vi "LocalHostServer.vi"() -> ()   [LabVIEW 2016]
uses:
  FTT/controls/SocketServerStates.ctl
panel:
  out "LocalHostCommState":bool
  out "Ch2":fxp<+/-,20,5>
  out "Ch1":fxp<+/-,20,5>
  out "error out":errorcluster
  in  "error in (no error)":errorcluster
  in  "stop":bool
  out "length":i32
  out "bytes written":i32
  out "bytes written 2":i32
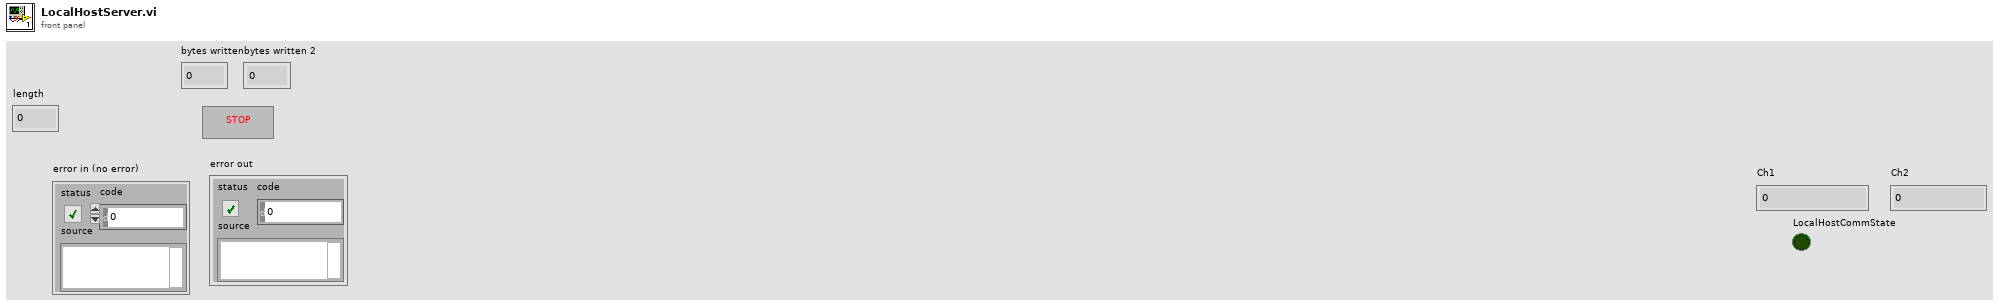
[diagram p1: front panel]
types:
  T1 = typedef "SocketServerStates.ctl" = enum16{"Wait", "SwitchState", "SingleUpdate", "ClosedLoop", "GetValues", "Exit"}
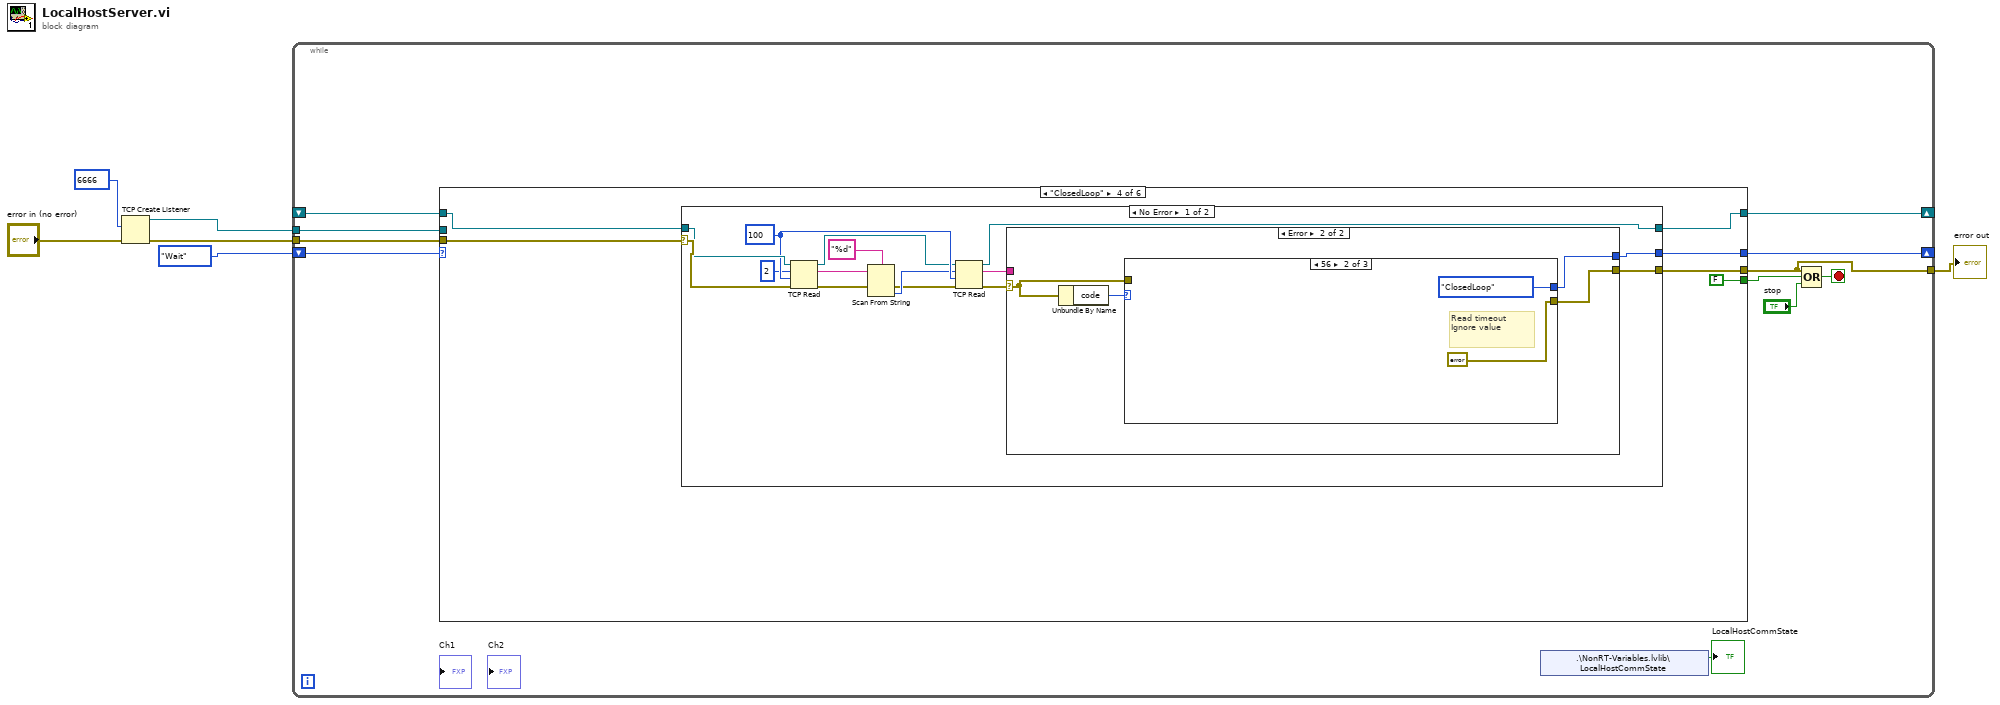
[diagram p0: block diagram]
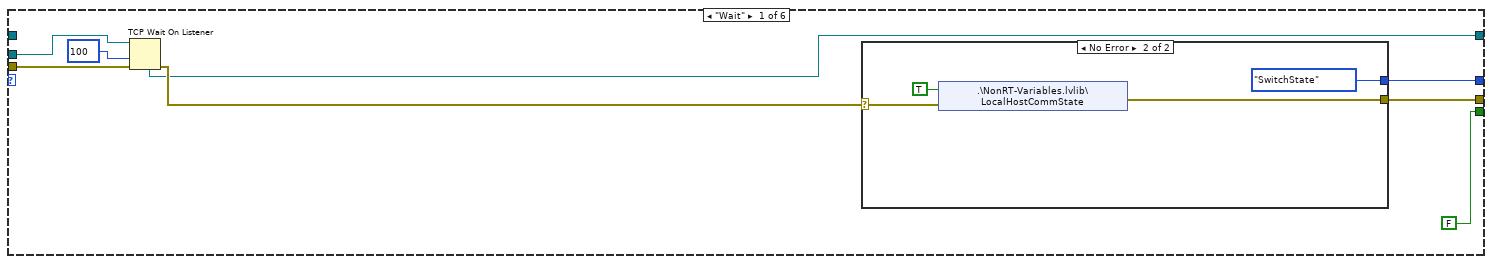
[diagram p2: hidden frame]
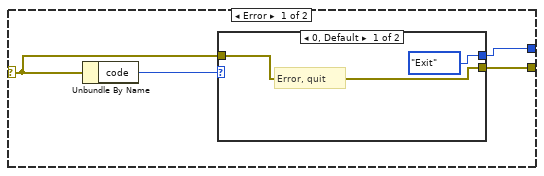
[diagram p3: hidden frame]
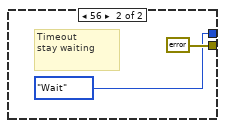
[diagram p4: hidden frame]
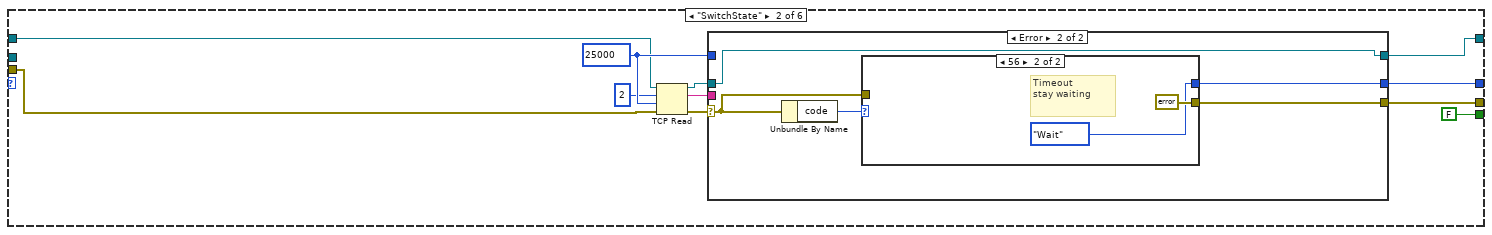
[diagram p5: hidden frame]
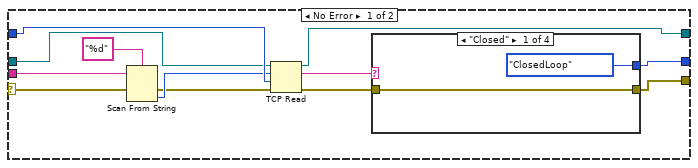
[diagram p6: hidden frame]
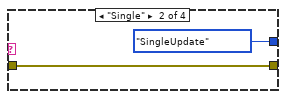
[diagram p7: hidden frame]
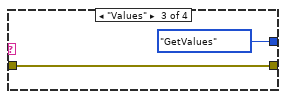
[diagram p8: hidden frame]
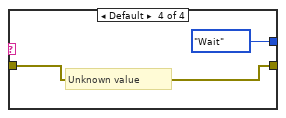
[diagram p9: hidden frame]
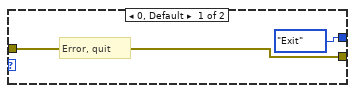
[diagram p10: hidden frame]
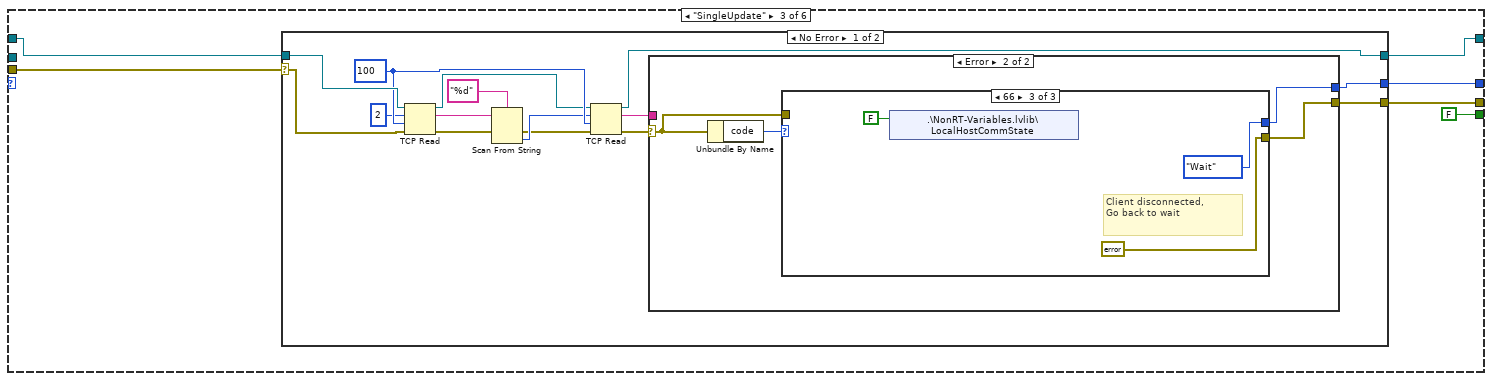
[diagram p11: hidden frame]
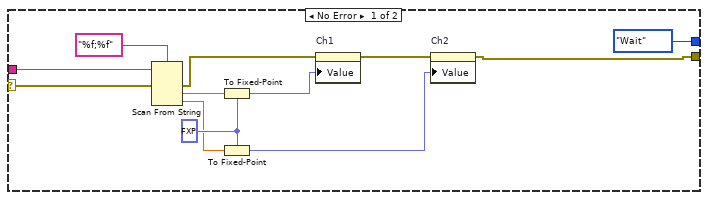
[diagram p12: hidden frame]
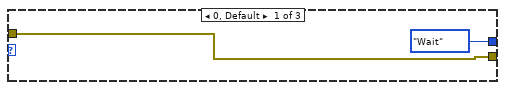
[diagram p13: hidden frame]
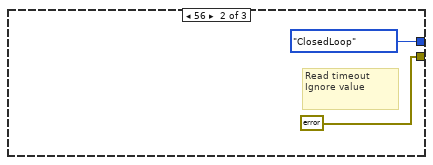
[diagram p14: hidden frame]
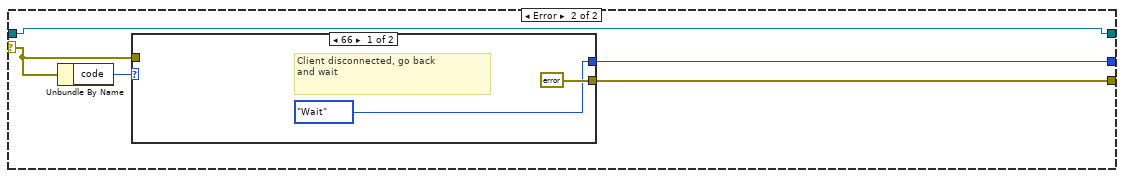
[diagram p15: hidden frame]
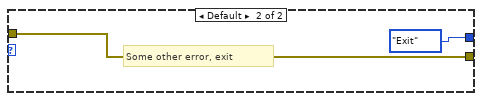
[diagram p16: hidden frame]
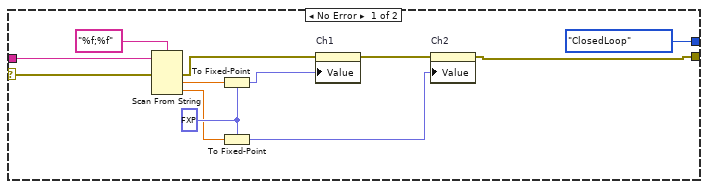
[diagram p17: hidden frame]
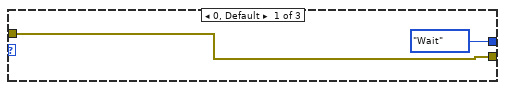
[diagram p18: hidden frame]
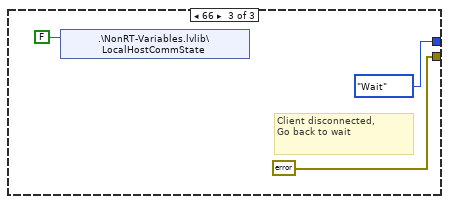
[diagram p19: hidden frame]
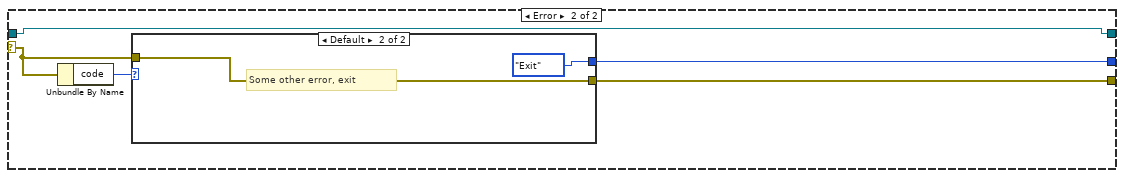
[diagram p20: hidden frame]
diagram:
  n1 = TCP Create Listener(8:"error in (no error)", 10:u16 6666 ("port")) -> (0:w3:errorcluster, 3:w5:refnum<k5>)  [unwired: 3 in, 1 out]
  n2 = while {
    tunnel: w5 -> [w17]
    tunnel: w3 -> [w11]
    shift-right: [w16] -> _
    shift-left: _ -> [w15]
    tunnel: [w10] -> w1
    shift-right: [w9] -> _
    shift-left: SocketServerStates."Wait" -> [w8]
    stop <- w13 stop-if-true
    n3 = case shown="\"ClosedLoop\"" w8 {
      tunnel: w11 -> [w24 w41 w83 w136 w185 w235]
      tunnel: w17 -> [w22 _ _ _ _ w236]
      tunnel: [w21 w47 w79 w135 w186 w234] -> w10
      tunnel: [w18 w48 w80 w134 w188 SocketServerStates."Exit"] -> w9
      tunnel: [w19 w39 w81 w132 w187 w237] -> w16
      tunnel: w15 -> [_ w40 w82 w133 w189 w237]
      tunnel: [FALSE FALSE FALSE FALSE FALSE TRUE] -> w12
      frame "Wait" {
        n4 = TCP Wait On Listener(8:w24, 9:100 ("timeout ms (wait forever: -1)"), 11:w22) -> (0:w23:errorcluster, 4:w19:refnum<k5>)  [unwired: 1 in, 3 out]
        n5 = case shown="No Error" w23 {
          selector: w23 -> [w27 w35]
          tunnel: [w28 w36] -> w21
          tunnel: [w26 SocketServerStates."SwitchState"] -> w18
          frame Error {
            n6 = Unbundle By Name(w27) -> ("code"=w29:i32)
            n7 = case shown="0, Default" w29 {
              tunnel: [w31 errorcluster {"status"=FALSE, "code"=0, "source"=""} ("error constant")] -> w28
              tunnel: w27 -> [w31 _]
              tunnel: [SocketServerStates."Exit" SocketServerStates."Wait"] -> w26
              frame 0, Default {
                # "Error, quit"
              }
              frame 56 {
                # "Timeout\nstay waiting"
              }
            }
          }
          frame No Error {
            n8 = shared-variable ".\\NonRT-Variables.lvlib\\LocalHostCommState"(TRUE ("FTTCommState"), error in=w35) -> (error out=w36:errorcluster)
          }
        }
      }
      frame "SwitchState" {
        w45 = 25000 ("timeout ms (25000)")
        n9 = TCP Read(connection ID=w40, bytes to read=2, error in (no error)=w41, 9:w45) -> (connection ID out=w43:refnum<k5>, data out=w44:string, error out=w38:errorcluster)  [unwired: 1 in]
        n10 = case shown="Error" w38 {
          selector: w38 -> [w49 w72]
          tunnel: [w60 w71] -> w48
          tunnel: [w59 w70] -> w47
          tunnel: w45 -> [w58 _]
          tunnel: w44 -> [w55 _]
          tunnel: w43 -> [w54 w69]
          tunnel: [w50 w69] -> w39
          frame No Error {
            n11 = Scan From String(format string="%d", input string=w55, error in=w49) -> (error out=w56:errorcluster, output 1=w57:i32)  [unwired: 2 in, 2 out]
            n12 = TCP Read(connection ID=w54, bytes to read=w57, error in (no error)=w56, 9:w58) -> (connection ID out=w50:refnum<k5>, data out=w51:string, error out=w52:errorcluster)  [unwired: 1 in]
            n13 = case shown="\"Closed\"" w51 {
              tunnel: [SocketServerStates."ClosedLoop" SocketServerStates."SingleUpdate" SocketServerStates."GetValues" SocketServerStates."Wait"] -> w60
              tunnel: w52 -> [w61 w63 w65 w68]
              tunnel: [w61 w63 w65 w68] -> w59
              frame "Closed" {
              }
              frame "Single" {
              }
              frame "Values" {
              }
              frame Default {
                # "Unknown value"
              }
            }
          }
          frame Error {
            n14 = Unbundle By Name(w72) -> ("code"=w73:i32)
            n15 = case shown="56" w73 {
              tunnel: [w75 errorcluster {"status"=FALSE, "code"=0, "source"=""} ("error constant")] -> w70
              tunnel: w72 -> [w75 _]
              tunnel: [SocketServerStates."Exit" SocketServerStates."Wait"] -> w71
              frame 0, Default {
                # "Error, quit"
              }
              frame 56 {
                # "Timeout\nstay waiting"
              }
            }
          }
        }
      }
      frame "SingleUpdate" {
        n16 = case shown="No Error" w83 {
          selector: w83 -> [w93 w125]
          tunnel: [w97 w124] -> w79
          tunnel: [w94 w123] -> w80
          tunnel: w82 -> [w92 w122]
          tunnel: [w95 w122] -> w81
          frame No Error {
            w91 = 100 ("timeout ms (25000)")
            n17 = TCP Read(connection ID=w92, bytes to read=2, error in (no error)=w93, 9:w91) -> (connection ID out=w86:refnum<k5>, data out=w87:string, error out=w90:errorcluster)  [unwired: 1 in]
            n18 = Scan From String(format string="%d", input string=w87, error in=w90) -> (error out=w88:errorcluster, output 1=w89:i32)  [unwired: 2 in, 2 out]
            n19 = TCP Read(connection ID=w86, bytes to read=w89, error in (no error)=w88, 9:w91) -> (connection ID out=w95:refnum<k5>, data out=w96:string, error out=w98:errorcluster)  [unwired: 1 in]
            n20 = case shown="Error" w98 {
              selector: w98 -> [w107 w113]
              tunnel: [w99 w112] -> w97
              tunnel: w96 -> [w109 _]
              tunnel: [SocketServerStates."Wait" w111] -> w94
              frame No Error {
                w108 = fxp<+/-,20,5> 0.0 ("fixed-point type")
                n21 = Scan From String(format string="%f;%f", input string=w109, error in=w107) -> (error out=w101:errorcluster, output 1=w106:dbl, output 2=w105:dbl)  [unwired: 3 in, 2 out]
                n22 = To Fixed-Point(fixed-point type=w108, number=w106) -> (fixed-point=w102:fxp<+/-,20,5>)
                n23 = To Fixed-Point(fixed-point type=w108, number=w105) -> (fixed-point=w103:fxp<+/-,20,5>)
                n24 = property on="Ch1" class="DigNum (strict)"(error in=w101, "Value"=w102) -> (error out=w100:errorcluster)  [unwired: 1 in, 1 out]
                n25 = property on="Ch2" class="DigNum (strict)"(error in=w100, "Value"=w103) -> (error out=w99:errorcluster)  [unwired: 1 in, 1 out]
              }
              frame Error {
                n26 = Unbundle By Name(w113) -> ("code"=w114:i32)
                n27 = case shown="66" w114 {
                  tunnel: w113 -> [w116 _ _]
                  tunnel: [w116 errorcluster {"status"=FALSE, "code"=0, "source"=""} ("error constant") errorcluster {"status"=FALSE, "code"=0, "source"=""} ("error constant")] -> w112
                  tunnel: [SocketServerStates."Wait" SocketServerStates."ClosedLoop" SocketServerStates."Wait"] -> w111
                  frame 0, Default {
                  }
                  frame 56 {
                    # "Read timeout\nIgnore value"
                  }
                  frame 66 {
                    # "Client disconnected,\nGo back to wait"
                    n28 = shared-variable ".\\NonRT-Variables.lvlib\\LocalHostCommState"(FALSE ("Cal. Mirror")) -> ()  [unwired: 1 in, 1 out]
                  }
                }
              }
            }
          }
          frame Error {
            n29 = Unbundle By Name(w125) -> ("code"=w126:i32)
            n30 = case shown="66" w126 {
              tunnel: w125 -> [_ w130]
              tunnel: [errorcluster {"status"=FALSE, "code"=0, "source"=""} ("error constant") w130] -> w124
              tunnel: [SocketServerStates."Wait" SocketServerStates."Exit"] -> w123
              frame 66 {
                # "Client disconnected, go back\nand wait"
              }
              frame Default {
                # "Some other error, exit"
              }
            }
          }
        }
      }
      frame "ClosedLoop" {
        n31 = case shown="No Error" w136 {
          selector: w136 -> [w146 w178]
          tunnel: [w150 w177] -> w135
          tunnel: [w147 w176] -> w134
          tunnel: w133 -> [w145 w175]
          tunnel: [w148 w175] -> w132
          frame No Error {
            w144 = 100 ("timeout ms (25000)")
            n32 = TCP Read(connection ID=w145, bytes to read=2, error in (no error)=w146, 9:w144) -> (connection ID out=w139:refnum<k5>, data out=w140:string, error out=w143:errorcluster)  [unwired: 1 in]
            n33 = Scan From String(format string="%d", input string=w140, error in=w143) -> (error out=w141:errorcluster, output 1=w142:i32)  [unwired: 2 in, 2 out]
            n34 = TCP Read(connection ID=w139, bytes to read=w142, error in (no error)=w141, 9:w144) -> (connection ID out=w148:refnum<k5>, data out=w149:string, error out=w151:errorcluster)  [unwired: 1 in]
            n35 = case shown="Error" w151 {
              selector: w151 -> [w160 w166]
              tunnel: [w152 w165] -> w150
              tunnel: w149 -> [w162 _]
              tunnel: [SocketServerStates."ClosedLoop" w164] -> w147
              frame No Error {
                w161 = fxp<+/-,20,5> 0.0 ("fixed-point type")
                n36 = Scan From String(format string="%f;%f", input string=w162, error in=w160) -> (error out=w154:errorcluster, output 1=w157:dbl, output 2=w158:dbl)  [unwired: 3 in, 2 out]
                n37 = To Fixed-Point(fixed-point type=w161, number=w157) -> (fixed-point=w156:fxp<+/-,20,5>)
                n38 = To Fixed-Point(fixed-point type=w161, number=w158) -> (fixed-point=w155:fxp<+/-,20,5>)
                n39 = property on="Ch1" class="DigNum (strict)"(error in=w154, "Value"=w156) -> (error out=w153:errorcluster)  [unwired: 1 in, 1 out]
                n40 = property on="Ch2" class="DigNum (strict)"(error in=w153, "Value"=w155) -> (error out=w152:errorcluster)  [unwired: 1 in, 1 out]
              }
              frame Error {
                n41 = Unbundle By Name(w166) -> ("code"=w167:i32)
                n42 = case shown="56" w167 {
                  tunnel: w166 -> [w169 _ _]
                  tunnel: [w169 errorcluster {"status"=FALSE, "code"=0, "source"=""} ("error constant") errorcluster {"status"=FALSE, "code"=0, "source"=""} ("error constant")] -> w165
                  tunnel: [SocketServerStates."Wait" SocketServerStates."ClosedLoop" SocketServerStates."Wait"] -> w164
                  frame 0, Default {
                  }
                  frame 56 {
                    # "Read timeout\nIgnore value"
                  }
                  frame 66 {
                    # "Client disconnected,\nGo back to wait"
                    n43 = shared-variable ".\\NonRT-Variables.lvlib\\LocalHostCommState"(FALSE ("Cal. Mirror")) -> ()  [unwired: 1 in, 1 out]
                  }
                }
              }
            }
          }
          frame Error {
            n44 = Unbundle By Name(w178) -> ("code"=w179:i32)
            n45 = case shown="Default" w179 {
              tunnel: w178 -> [_ w183]
              tunnel: [errorcluster {"status"=FALSE, "code"=0, "source"=""} ("error constant") w183] -> w177
              tunnel: [SocketServerStates."Wait" SocketServerStates."Exit"] -> w176
              frame 66 {
                # "Client disconnected, go back\nand wait"
              }
              frame Default {
                # "Some other error, exit"
              }
            }
          }
        }
      }
      frame "GetValues" {
        n46 = case shown="Error" w185 {
          selector: w185 -> [w191 w226]
          tunnel: [w192 w225] -> w186
          tunnel: [w193 w224] -> w188
          tunnel: w189 -> [w205 w223]
          tunnel: [w201 w223] -> w187
          frame No Error {
            w190 = sgl 0.0 ("number")
            w208 = "" ("initial string")
            w200 = 25000 ("timeout ms (25000)")
            n47 = To Single Precision Float(number=w190) -> (single precision float=w211:sgl)
            n48 = To Single Precision Float(number=w190) -> (single precision float=w210:sgl)
            n49 = Format Into String(format string="%f;%f", initial string=w208, error in=w191, w211, w210) -> (resulting string=w199:string, error out=w207:errorcluster)
            n50 = String Length(string=w199) -> (length=w209:i32)
            n51 = Format Into String(format string="%2d", initial string=w208, error in=w207, w209) -> (resulting string=w198:string, error out=w204:errorcluster)
            n52 = String Length(string=w198) -> (length=→"length":i32)
            n53 = TCP Write(connection ID=w205, data in=w198, error in (no error)=w204, 9:w200) -> (connection ID out=w202:refnum<k5>, bytes written=→"bytes written":i32, error out=w203:errorcluster)
            n54 = TCP Write(connection ID=w202, data in=w199, error in (no error)=w203, 9:w200) -> (connection ID out=w201:refnum<k5>, bytes written=→"bytes written 2":i32, error out=w194:errorcluster)
            n55 = case shown="No Error" w194 {
              selector: w194 -> [w213 w217]
              tunnel: [SocketServerStates."Wait" w218] -> w193
              tunnel: [w213 w215] -> w192
              frame No Error {
              }
              frame Error {
                n56 = Unbundle By Name(w217) -> ("code"=w216:i32)
                n57 = case shown="66" w216 {
                  tunnel: [SocketServerStates."Exit" SocketServerStates."Wait"] -> w218
                  tunnel: [errorcluster {"status"=FALSE, "code"=0, "source"=""} ("error constant") errorcluster {"status"=FALSE, "code"=0, "source"=""} ("error constant")] -> w215
                  frame 0, Default {
                  }
                  frame 66 {
                    # "Timeout"
                  }
                }
              }
            }
          }
          frame Error {
            n58 = Unbundle By Name(w226) -> ("code"=w227:i32)
            n59 = case shown="66" w227 {
              tunnel: w226 -> [_ _]
              tunnel: [errorcluster {"status"=FALSE, "code"=0, "source"=""} ("error constant") errorcluster {"status"=FALSE, "code"=0, "source"=""} ("error constant")] -> w225
              tunnel: [SocketServerStates."Wait" SocketServerStates."Exit"] -> w224
              frame 66 {
                # "Client disconnected, go back\nand wait"
              }
              frame Default {
                # "Some other error, exit"
              }
            }
          }
        }
      }
      frame "Exit", Default {
        n60 = TCP Close Connection(connection ID=w236, error in (no error)=w235) -> (error out=w234:errorcluster)  [unwired: 1 in, 1 out]
      }
    }
    n61 = shared-variable ".\\NonRT-Variables.lvlib\\LocalHostCommState"() -> (→"LocalHostCommState":bool)  [unwired: 1 in, 1 out]
    n62 = Compound Arithmetic op=OR(w10, w12, "stop") -> (w13:bool)
  }
  "error out" <- w1
